vi "library_path.vi"() -> (2 "library path":path)   [LabVIEW 2020, in "Nominal Streaming.lvlib"]
uses:
  Nominal Streaming.lvlib
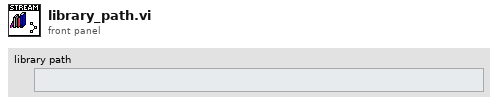
[diagram p1: front panel]
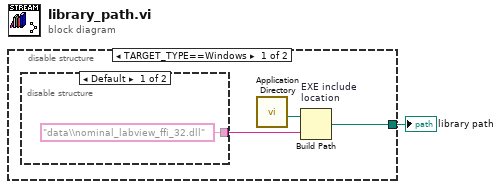
[diagram p0: block diagram]
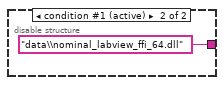
[diagram p2: hidden frame]
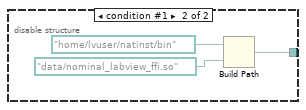
[diagram p3: hidden frame]
diagram:
  n1 = disable-structure shown="TARGET_TYPE==Windows" {
    disable-tunnel: [w2 w7] -> w1
    frame condition #0 (active) {
      n2 = disable-structure shown="Default" {
        disable-tunnel: ["data\\nominal_labview_ffi_32.dll" ("name or relative path") "data\\nominal_labview_ffi_64.dll" ("name or relative path")] -> w4
        frame condition #0 {
        }
        frame condition #1 (active) {
        }
      }
      n3 = call <vilib>:"Application Directory.vi"() -> ("Application Directory"=w3:path)
      n4 = Build Path "EXE include\nlocation"(base path=w3, name or relative path=w4) -> (appended path=w2:path)
    }
    frame condition #1 {
      n5 = Build Path(base path=path "home/lvuser/natinst/bin" ("path"), name or relative path=path "data/nominal_labview_ffi.so" ("path")) -> (appended path=w7:path)
    }
  }
  "library path" <- w1
